vi "Parse CSV Line.vi"(8 "error in":errorcluster, 11 "Input String":string) -> (0 "error out":errorcluster, 3 "values":dbl[](array[numeric]))   [LabVIEW 2023]
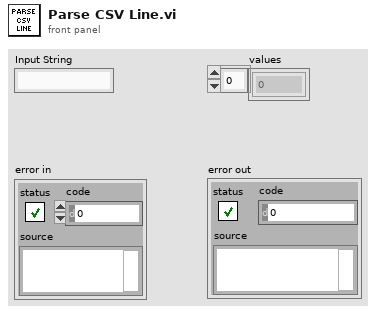
[diagram p1: front panel]
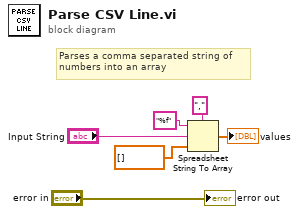
[diagram p0: block diagram]
diagram:
  # "Parses a comma separated string of \nnumbers into an array"
  n1 = Spreadsheet String To Array(delimiter (Tab)=",", format string="%f", spreadsheet string="Input String", array type (2D Dbl)=dbl[] []) -> (array=→"values":dbl[])
  "error out" <- "error in"
